vi "F4.vi"(8 "error in (no error)":errorcluster, 9 "data":u8[](array[numeric]), 10 "function":u8, 11 "device data model in":refnum<class "Standard Data Model.lvclass">) -> (0 "error out":errorcluster, 1 "data return":u8[](array[numeric]), 2 "function return":u8, 3 "device data model out":refnum<class "Standard Data Model.lvclass">)   [LabVIEW 2017, in "SubVIs.lvlib" / "Standard Data Model.lvclass"]
doc: "Executes function code 4"
uses:
  <vilib>/Modbus/subvis/Data and Functions/Standard Data Model/Standard Data Model.lvclass
  <vilib>/Modbus/subvis/SubVIs.lvlib
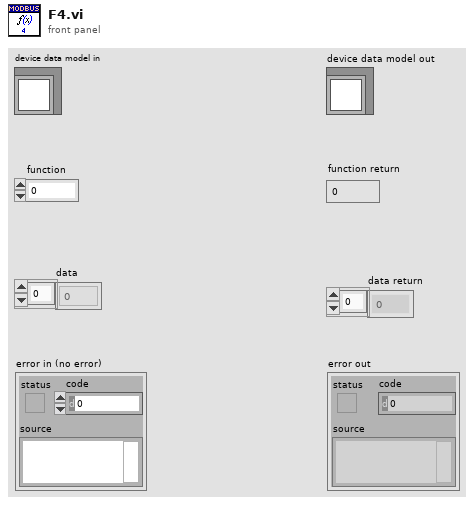
[diagram p1: front panel]
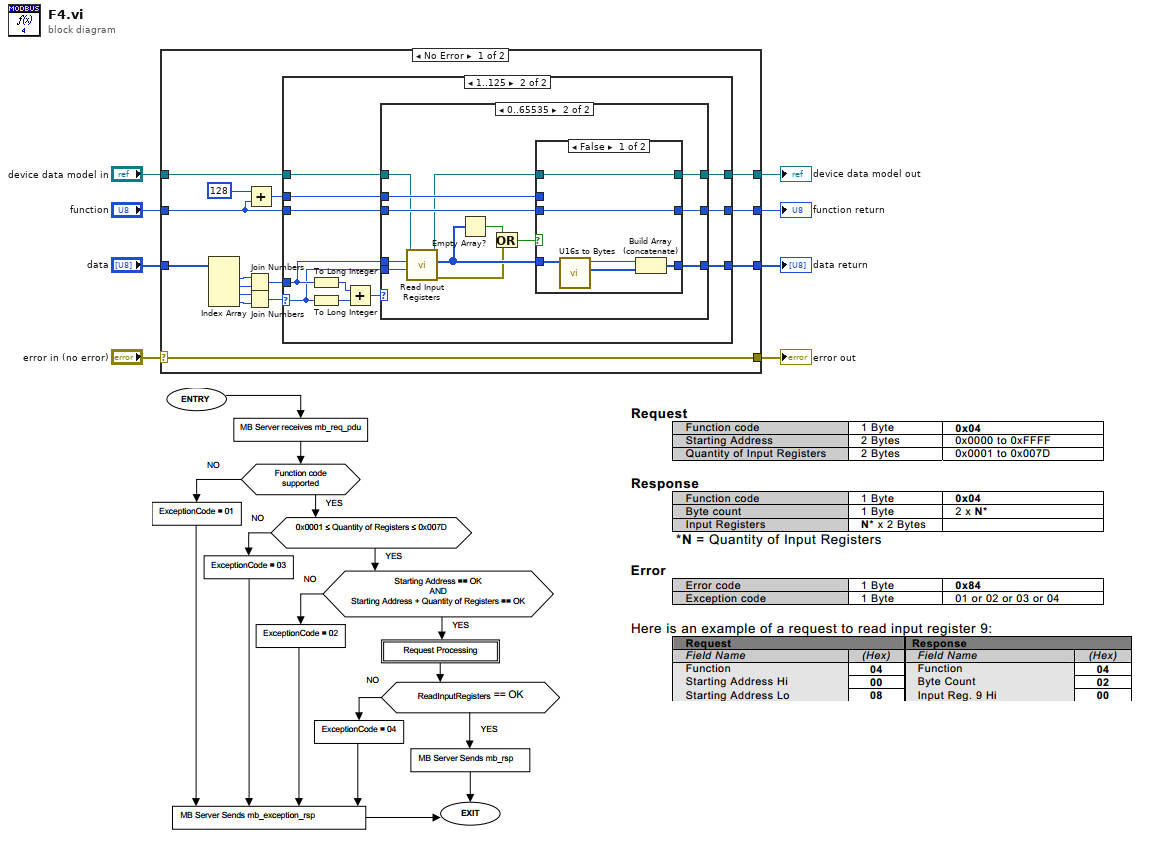
[diagram p0: block diagram]
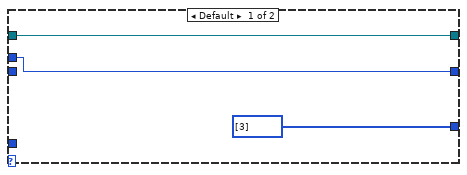
[diagram p2: hidden frame]
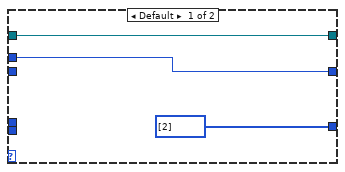
[diagram p3: hidden frame]
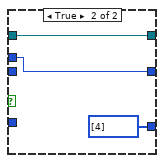
[diagram p4: hidden frame]
diagram:
  n1 = case shown="No Error" "error in (no error)" {
    selector: "error in (no error)" -> [w23 w66]
    tunnel: [w23 w66] -> w7
    tunnel: [w16 w65] -> w5
    tunnel: "device data model in" -> [w15 w65]
    tunnel: "function" -> [w12 w64]
    tunnel: "data" -> [w18 w63]
    tunnel: [w11 w64] -> w2
    tunnel: [w10 w63] -> w1
    frame No Error {
      n2 = Index Array(array=w18) -> (element #1=w21:u8, element #2=w22:u8, element #3=w20:u8, element #4=w19:u8)  [unwired: 4 in]
      n3 = Join Numbers(hi=w21, lo=w22) -> ((hi.lo)=w9:u16)
      n4 = Join Numbers(hi=w20, lo=w19) -> ((hi.lo)=w17:u16)
      n5 = Add(x=u8 128, y=w12) -> (x+y=w13:u8)
      n6 = case shown="1..125" w17 {
        selector: w17 -> [_ w33]
        tunnel: [w26 w32] -> w16
        tunnel: w15 -> [w26 w31]
        tunnel: w13 -> [w25 w30]
        tunnel: w12 -> [_ w28]
        tunnel: [w25 w29] -> w11
        tunnel: [u8[] [3] ("Data Return") w27] -> w10
        tunnel: w9 -> [_ w34]
        frame Default {
        }
        frame 1..125 {
          n7 = To Long Integer(number=w34) -> (32bit integer=w37:i32)
          n8 = To Long Integer(number=w33) -> (32bit integer=w36:i32)
          n9 = Add(x=w37, y=w36) -> (x+y=w35:i32)
          n10 = case shown="0..65535" w35 {
            tunnel: w34 -> [_ w43]
            tunnel: w33 -> [_ w44]
            tunnel: [w40 w52] -> w32
            tunnel: w31 -> [w40 w47]
            tunnel: w30 -> [w39 w51]
            tunnel: [w39 w49] -> w29
            tunnel: w28 -> [_ w50]
            tunnel: [u8[] [2] ("Data Return") w48] -> w27
            frame Default {
            }
            frame 0..65535 {
              n11 = call-dynamic "Read Input Registers.vi"("number of registers"=w44, "starting address"=w43, "device data model in"=w47) -> ("error out"=w41:errorcluster, "data"=w45:u16[], "device data model out"=w46:refnum<class "Standard Data Model.lvclass">)  [unwired: 6 in]
              n12 = Empty Array?(array=w45) -> (empty?=w42:bool)
              n13 = Or(x=w42, y=w41) -> (x .or. y?=w53:bool)
              n14 = case shown="False" w53 {
                tunnel: w46 -> [w59 w62]
                tunnel: [w59 w62] -> w52
                tunnel: w51 -> [_ w61]
                tunnel: w50 -> [w58 _]
                tunnel: [w58 w61] -> w49
                tunnel: w45 -> [w55 _]
                tunnel: [w57 u8[] [4]] -> w48
                frame False {
                  n15 = call <vilib>:"U16s to Bytes.vi"("registers"=w55) -> ("bytes"=w56:u8[], "count"=w54:u8)  [unwired: 9 in]
                  n16 = Build Array (concatenate)(w54, w56) -> (w57:u8[])
                }
                frame True {
                }
              }
            }
          }
        }
      }
    }
    frame Error {
    }
  }
  "error out" <- w7
  "device data model out" <- w5
  "data return" <- w1
  "function return" <- w2
